vi "GSM DATA SOCKET.vi"() -> ()   [LabVIEW 2013]
panel:
  out "URL Selected":bool
  out "error out":errorcluster
  out "Selected URL":string
  in  "Stop":bool
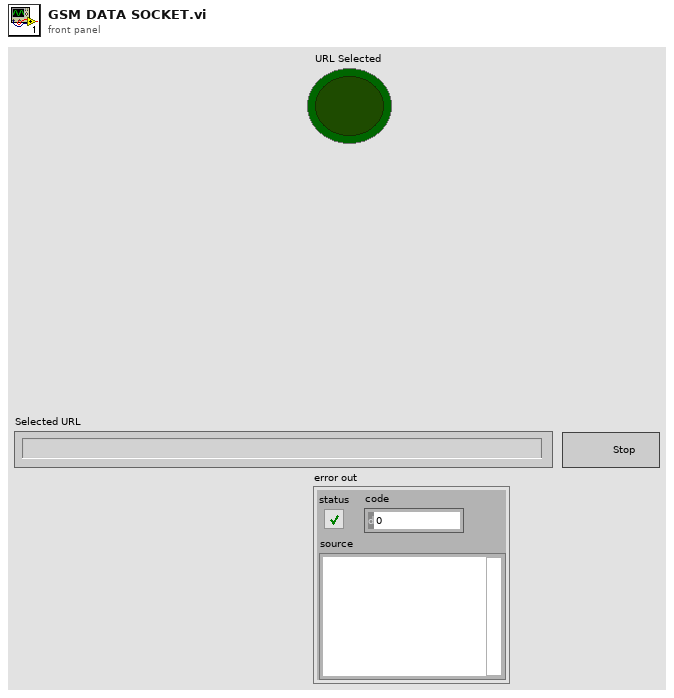
[diagram p1: front panel]
types:
  T1 = enum16{"Read", "Write", "ReadWrite", "BufferedRead", "BufferedReadWrite"}
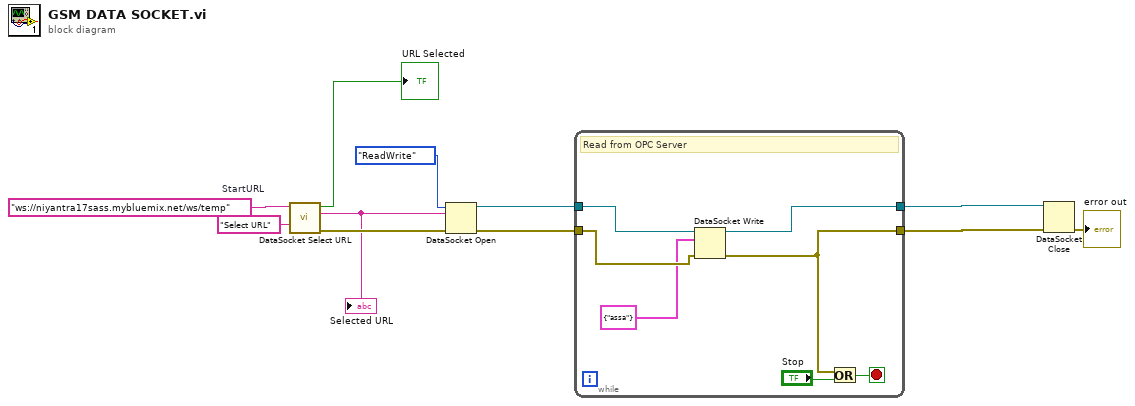
[diagram p0: block diagram]
diagram:
  w7 = "ws://niyantra17sass.mybluemix.net/ws/temp"  # StartURL
  n1 = call <vilib>:"DataSocket Select URL.vi"("Title (Select URL)"="Select URL", "StartURL (empty)"=w7) -> ("error out"=w6:errorcluster, "URL"=w4:string, "URL Selected"=→"URL Selected":bool)  [unwired: 1 in, 6 out]
  "Selected URL" <- w4
  n2 = DataSocket Open(8:w6, 10:T1."ReadWrite" ("mode"), 11:w4) -> (0:w9:errorcluster, 3:w11:refnum<k13>)  [unwired: 1 out]
  n3 = while {
    tunnel: [w13] -> w8
    tunnel: w9 -> [w14]
    tunnel: [w15] -> w10
    tunnel: w11 -> [w16]
    stop <- w18 stop-if-true
    # "Read from OPC Server"
    n4 = DataSocket Write(8:w14, 10:cluster{"String":string} {"String"="assa"} ("data"), 11:w16) -> (0:w13:errorcluster, 3:w15:refnum<k13>)  [unwired: 1 in, 1 out]
    n5 = Or(x=w13, y="Stop") -> (x .or. y?=w18:bool)
  }
  n6 = DataSocket Close(8:w8, 11:w10) -> (0:→"error out":errorcluster)  [unwired: 2 out]
